vi "Get Lines.vi"(0 "task name":refnum<k21>, 5 "channel list":string) -> (4 "lines":tag)   [LabVIEW 2021, in "DAQmxMeasurement1.lvlib"]
uses:
  DAQmxMeasurement1.lvlib
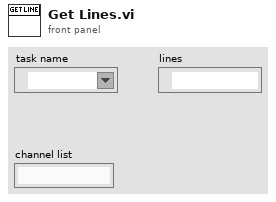
[diagram p1: front panel]
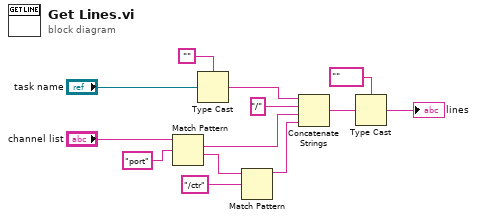
[diagram p0: block diagram]
diagram:
  n1 = Match Pattern(string="channel list", regular expression="port") -> (match substring=w10:string, after substring=w11:string)  [unwired: 1 in, 2 out]
  n2 = Type Cast(type="", x="task name") -> (*(type *) &x=w2:string)
  n3 = Match Pattern(string=w11, regular expression="/ctr") -> (before substring=w13:string)  [unwired: 1 in, 3 out]
  n4 = Concatenate Strings(w2, "/" ("string"), w10, w13) -> (w6:string)
  n5 = Type Cast(type=tag "" ("lines"), x=w6) -> (*(type *) &x=→"lines":tag)
